vi "FRCts20_Backend_Comment_PUT.vi"(6 "Message Attributes":T4, 8 "error in (no error)":errorcluster, 10 "Data":string, 11 "Engine_Refnums":T1) -> (0 "error out":errorcluster)   [LabVIEW 2013, in "FRCts20_Backend_Engine.lvlib"]
doc: "Marks a comment as a solution (or unmarks), called by the Comment API. Expects a comment index and a boolean."
uses:
  FRCts20_Backend_Engine.lvlib
  Dependencies/Keyed Array/KeyedArray.ctl
  FRCts20_Backend_EngineRefnums.ctl
  INI_Accessor/FRCts20_Backend_INI Controller.lvclass
  Dependencies/AMC/_SubVIs/TypeDefs/Message Queue.ctl
  Dependencies/AMC/_SubVIs/TypeDefs/Message.ctl
  <vilib>/addons/database/Connection.llb/Conn ObjectReference.ctl
  FRCts20_Backend_FGVOperation.ctl
  FRCts20_Backend_API/FRCts20_Backend_API_Note.ctl
  FRCts20_Backend_API/FRCts20_Backend_API.lvlib
  Dependencies/Keyed Array/Tools_KeyedArray.lvlib
  Dependencies/AMC/AMC.lvlib
  <vilib>/addons/database/NI_Database_API.lvlib
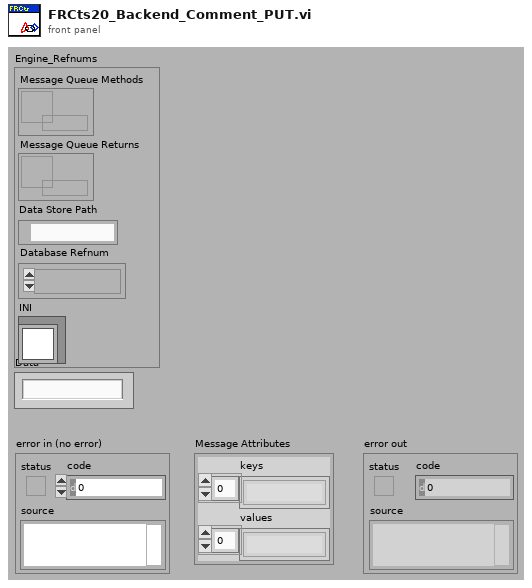
[diagram p1: front panel]
types:
  T1 = typedef "FRCts20_Backend_Engine.lvlib/FRCts20_Backend_EngineRefnums.ctl" = cluster{"Message Queue Methods":T2, "Message Queue Returns":T2, "Data Store Path":path, "Database Refnum":T3, "INI":refnum<class "FRCts20_Backend_INI Controller.lvclass">}
  T2 = typedef "AMC.lvlib/Message Queue.ctl" = refnum<queue>
  T3 = typedef "NI_Database_API.lvlib/Conn ObjectReference.ctl" = refnum<k1>
  T4 = typedef "Tools_KeyedArray.lvlib/KeyedArray.ctl" = cluster{"keys":string[], "values":string[]}
  T5 = typedef "FRCts20_Backend_API.lvlib/FRCts20_Backend_API_Note.ctl" = cluster{"Note Index":u32, "Request Index":u32, "Author":string, "Time Entered":timestamp, "Text":string, "Solution":bool, "APIReturn":string}
  T6 = typedef "FRCts20_Backend_Engine.lvlib/FRCts20_Backend_FGVOperation.ctl" = enum16{"Initialize", "EnqueueMessage", "EnqueueDataReturn", "FlushMessage", "FlushDataReturn"}
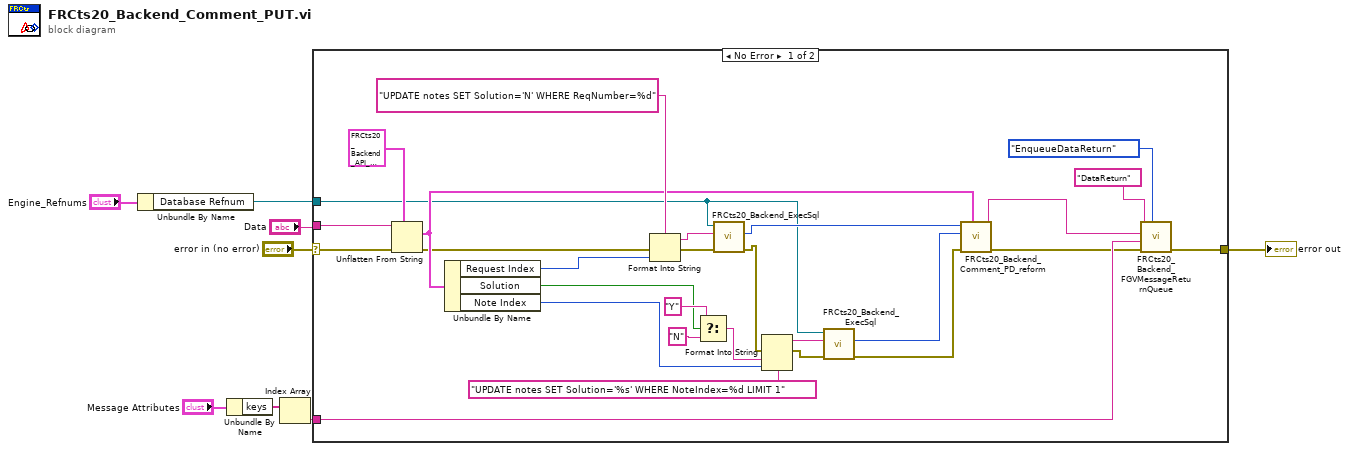
[diagram p0: block diagram]
diagram:
  n1 = Unbundle By Name("Engine_Refnums") -> ("Database Refnum"=w5:T3)
  n2 = Unbundle By Name("Message Attributes") -> ("keys"=w2:string[])
  n3 = Index Array(array=w2) -> (element=w1:string)  [unwired: 1 in]
  n4 = case shown="No Error" "error in (no error)" {
    selector: "error in (no error)" -> [w33 w37]
    tunnel: [w36 w37] -> w7
    tunnel: w5 -> [w11 _]
    tunnel: "Data" -> [w34 _]
    tunnel: w1 -> [w35 _]
    frame No Error {
      n5 = Unflatten From String(type=T5 {"Note Index"=0, "Request Index"=0, "Author"="", "Time Entered"=timestamp(0 s since 1904-01-01), "Text"="", "Solution"=FALSE, "APIReturn"=""} ("Note"), binary string=w34, error in (no error)=w33) -> (value=w20:T5, error out=w18:errorcluster)  [unwired: 2 in, 1 out]
      n6 = Unbundle By Name(w20) -> ("Request Index"=w19:u32, "Solution"=w24:bool, "Note Index"=w15:u32)
      n7 = Format Into String(format string="UPDATE notes SET Solution='N' WHERE ReqNumber=%d", error in=w18, w19) -> (resulting string=w22:string, error out=w23:errorcluster)  [unwired: 1 in]
      n8 = Select(t="Y", s=w24, f="N") -> (s? t:f=w16:string)
      n9 = call "FRCts20_Backend_ExecSql.vi"("error in (no error)"=w23, "format string"=w22, "Refnum in"=w11) -> ("error out"=w10:errorcluster, "rows affected"=w21:i32)  [unwired: 6 in, 1 out]
      n10 = Format Into String(format string="UPDATE notes SET Solution='%s' WHERE NoteIndex=%d LIMIT 1", error in=w10, w16, w15) -> (resulting string=w14:string, error out=w13:errorcluster)  [unwired: 1 in]
      n11 = call "FRCts20_Backend_ExecSql.vi"("error in (no error)"=w13, "format string"=w14, "Refnum in"=w11) -> ("error out"=w9:errorcluster, "rows affected"=w12:i32)  [unwired: 6 in, 1 out]
      n12 = call "FRCts20_Backend_Comment_PD_reform.vi"("Note"=w20, "error in (no error)"=w9, "rows affected 2"=w12, "rows affected"=w21) -> ("error out"=w28:errorcluster, "data string"=w29:string)  [unwired: 6 in]
      n13 = call "FRCts20_Backend_FGVMessageReturnQueue.vi"("Operation"=FRCts20_Backend_FGVOperation."EnqueueDataReturn", "error in (no error)"=w28, "Key"=w35, "Message Value"=w29, "Message Name"="DataReturn") -> ("error out"=w36:errorcluster)  [unwired: 5 in, 1 out]
    }
    frame Error {
    }
  }
  "error out" <- w7
